vi "SetConfigurationManager.vi"(7 "ConfigManager in":refnum<class "ConfigManager.lvclass">, 10 "error in (no error)":errorcluster, 11 "vi reference in":refnum<vi>) -> (2 "error out":errorcluster, 3 "vi reference out":refnum<vi>)   [LabVIEW 2014, in "ConfigurableQMH.lvlib"]
uses:
  <vilib>/LabVIEW Open Source/Configuration Manager/Manager/ConfigManager.lvclass
  ConfigurableQMH.lvlib
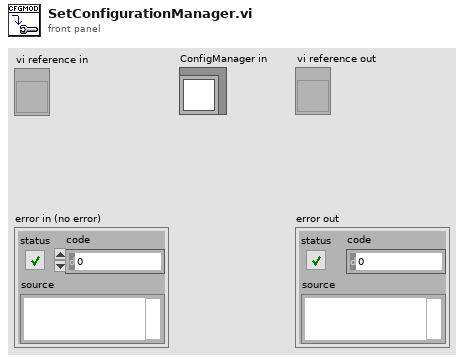
[diagram p1: front panel]
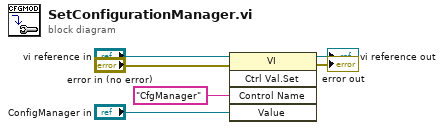
[diagram p0: block diagram]
diagram:
  n1 = invoke class="VI" method="Ctrl Val.Set"(reference="vi reference in", error in="error in (no error)", "Control Name"="CfgManager", "Value"="ConfigManager in") -> (reference out=→"vi reference out":refnum<vi>, error out=→"error out":errorcluster)  [unwired: 1 in, 3 out]
